vi "Getting Started - External Memory (Host).vi"() -> ()   [LabVIEW 2023]
doc: "This Host vi controls the data the flows into and out of the different external memory access methods on the FPGA."
uses:
  <vilib>/userDefined/Silver/nirio_resource_slv.ctl
  <vilib>/FPGAPlugInAG/PXIe-7966R/niLvFpga_Open_PXIe-7966R.vi
  <vilib>/rvi/interface/common/dynamic/niFpgaDynamicAddResources.vi
  <vilib>/Utility/error.llb/Error Cluster From Error Code.vi
  <vilib>/rvi/errors/niLvFpgaAdjustHostInterfaceError.vi
  <vilib>/FPGAPlugInAG/Dynamic/niLvFpga_Close_Dynamic.vi
  <vilib>/rvi/interface/nirviOpenFPGA/nirviOpenFPGA.xnode
  FPGA Bitfiles/Ext_Mem 7966R.lvbitx
  <vilib>/rvi/interface/nirviReadWriteControl/nirviReadWriteControl.xnode
  <vilib>/rvi/interface/nirviMethod/nirviMethod.xnode
  <vilib>/rvi/interface/nirviCloseFPGA/nirviCloseFPGA.xnode
  <vilib>/rvi/interface/Simulation/niFpgaSimulationCallBeginRW.vi
  <vilib>/rvi/errors/niLvFpgaMergeErrorWithErrorCode.vi
  NiFpgaLv.dll
  <vilib>/FPGAPlugInAG/Dynamic/niLvFpga_WriteFifo_Dynamic.vi
  <vilib>/FPGAPlugInAG/Dynamic/niLvFpga_ReadFifo_Dynamic.vi
panel:
  in  "Tab Control":T1(tab)
  in  "Memory Primitive - Write Address":u32
  in  "Memory Primitive - Write Data":u64
  in  "Memory Primitive - Write Valid":bool
  in  "Memory Primitive - Request Address":u32
  in  "Memory Primitive - Request Valid":bool
  out "Memory Primitive- Retrieved Data":u64
  out "Memory IDL - Retrieved Data":u64[](array[numeric])
  in  "Memory IDL - write grant time (clocks)":u16=100
  in  "Memory IDL - read grant time (clocks)":u16=100
  in  "Memory IDL - Write Data":u64[](array[numeric])
  in  "Memory IDL - Request Address":u32
  in  "Memory IDL - Request Valid":bool
  in  "Memory IDL - Write Valid":bool
  in  "Memory IDL - Write Address":u32
  in  "DRAM FIFO - Write Valid":bool
  in  "DRAM FIFO - write grant time (clocks)":u16=100
  in  "DRAM FIFO - read grant time (clocks)":u16=100
  out "DRAM FIFO Status":T2
  in  "DRAM FIFO - Write Data":u32[](array[numeric])
  out "DRAM FIFO - Retrieved Data":u32[](array[numeric])
  in  "Stop Button":bool
  in  "RIO Device":T3
  # "Overview: Demonstratethe different methods vailable for DRAM access on a FlexRIO FPGA Module.\nRequirements: LabVIEW FPGA Module, FlexRIO\nInstructions: \n 1. On the block diagram, configure the Open FPGA VI Reference function. \n 2. Return to the front panel and specify a valid RIO Device.\n 3. Run the VI \n 4. Select a tab and specify the value of Write Data  and Write address if applicable then click Write Valid.\n 5. Specify a Request Address if applicable and click Request Valid\n 6. (optional) Change the write/read grant time to zero for the read or write and observe access behavior"
  # "Note: 795x targets can read and write only the 0th element of the Write or Retrieved Data array. 796x targets the first two elements."
  # "Note: 795x targets can read and write only the first two element of the Write or Retrieved Data array.  The 796x the first four. The 797x all eight."
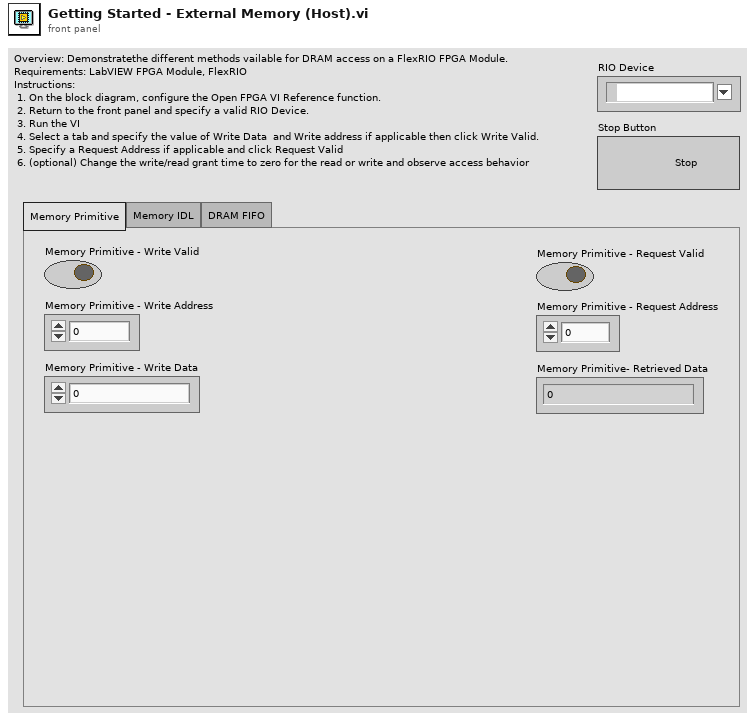
[diagram p1: front panel]
types:
  T1 = enum32{"Memory Primitive", "Memory IDL", "DRAM FIFO"}
  T2 = cluster{"Elements in To DRAM Queue":u32, "Elements in From DRAM Queue":u32, "Elements in DRAM":u32, "DRAM Full":bool, "DRAM Empty":bool}
  T3 = typedef "nirio_resource_slv.ctl" = tag
  T4 = cluster{"elements in 'to DRAM queue'":u32, "elements in 'from DRAM queue'":u32, "elements in DRAM":u32, "DRAM full":bool, "DRAM empty":bool}
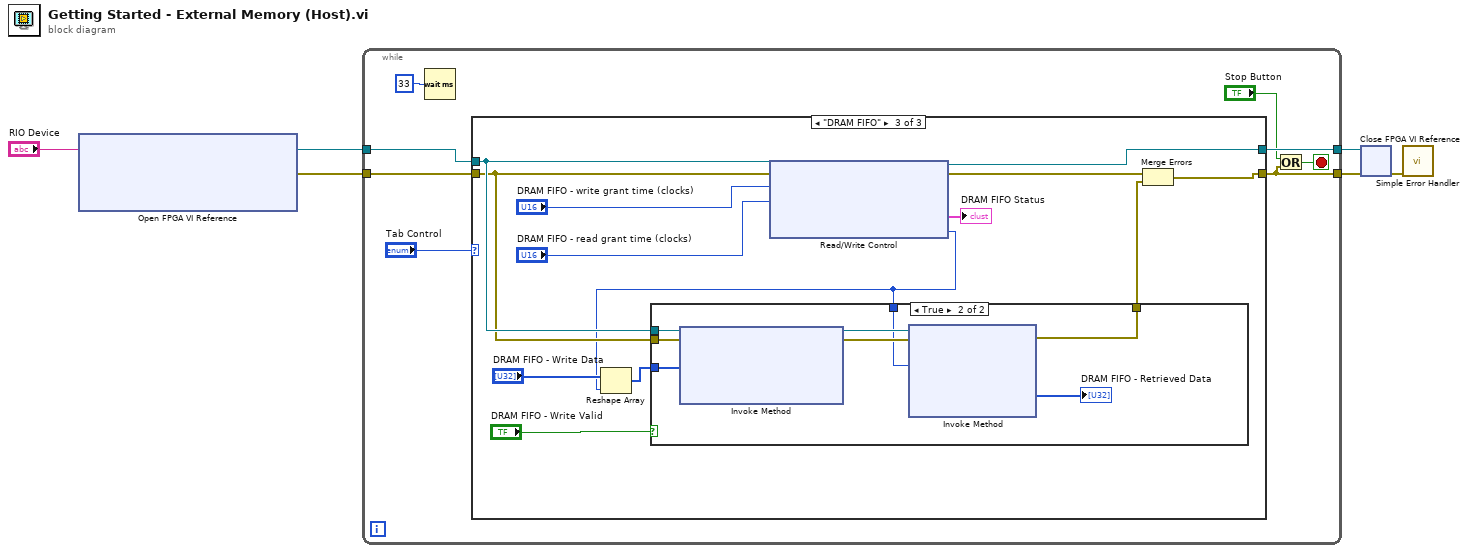
[diagram p0: block diagram]
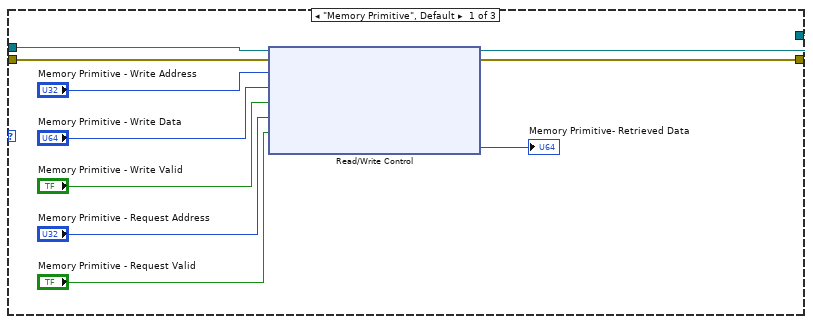
[diagram p2: hidden frame]
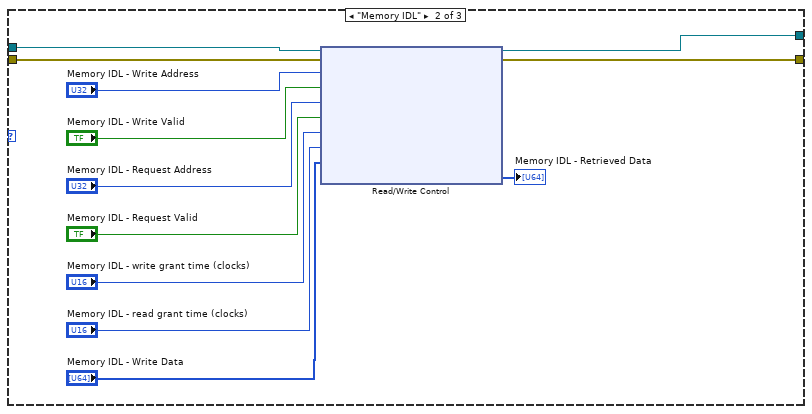
[diagram p3: hidden frame]
diagram:
  n1 = xnode "Open FPGA VI Reference"("resource name"="RIO Device") -> ("FPGA VI Reference Out"=w5:refnum<k20>, "error out"=w4:errorcluster)  [unwired: 1 in]
  n2 = while {
    tunnel: w5 -> [w14]
    tunnel: w4 -> [w12]
    tunnel: [w10] -> w2
    tunnel: [w13] -> w1
    stop <- w11 stop-if-true
    n3 = Wait (ms)(milliseconds to wait=u32 33) -> ()  [unwired: 1 out]
    n4 = case shown="\"DRAM FIFO\"" "Tab Control" {
      tunnel: w14 -> [w24 w36 w45]
      tunnel: [w23 w34 w49] -> w13
      tunnel: w12 -> [w22 w35 w44]
      tunnel: [w21 w33 w41] -> w10
      frame "Memory Primitive", Default {
        n5 = xnode "Read/Write Control"("FPGA VI Reference In"=w24, "error in"=w22, "Memory Primitive - Write Address"="Memory Primitive - Write Address", "Memory Primitive - Write Data"="Memory Primitive - Write Data", "Memory Primitive - Write Valid"="Memory Primitive - Write Valid", "Memory Primitive - Request Address"="Memory Primitive - Request Address", "Memory Primitive - Request Valid"="Memory Primitive - Request Valid") -> ("FPGA VI Reference Out"=w23:refnum<k20>, "error out"=w21:errorcluster, "Memory Primitive - Retrieved Data"=→"Memory Primitive- Retrieved Data":u64)
      }
      frame "Memory IDL" {
        n6 = xnode "Read/Write Control"("FPGA VI Reference In"=w36, "error in"=w35, "Memory IDL - Write Address"="Memory IDL - Write Address", "Memory IDL - Write Valid"="Memory IDL - Write Valid", "Memory IDL - Request Address"="Memory IDL - Request Address", "Memory IDL - Request Valid"="Memory IDL - Request Valid", "Memory IDL - write grant time"="Memory IDL - write grant time (clocks)", "Memory IDL - read grant time"="Memory IDL - read grant time (clocks)", "Memory IDL - Write Data"="Memory IDL - Write Data") -> ("FPGA VI Reference Out"=w34:refnum<k20>, "error out"=w33:errorcluster, "Memory IDL - Retrieved Data"=→"Memory IDL - Retrieved Data":u64[])
      }
      frame "DRAM FIFO" {
        n7 = xnode "Read/Write Control"("FPGA VI Reference In"=w45, "error in"=w44, "Memory IDL - write grant time"="DRAM FIFO - write grant time (clocks)", "Memory IDL - read grant time"="DRAM FIFO - read grant time (clocks)") -> ("FPGA VI Reference Out"=w49:refnum<k20>, "error out"=w42:errorcluster, "DRAM FIFO Status"=→"DRAM FIFO Status":T4, "elements per valid output"=w37:i32)
        n8 = Reshape Array("DRAM FIFO - Write Data", w37) -> (w38:u32[])
        n9 = case shown="True" "DRAM FIFO - Write Valid" {
          tunnel: w45 -> [_ w58]
          tunnel: w44 -> [w50 w57]
          tunnel: w38 -> [_ w56]
          tunnel: [w50 w52] -> w40
          tunnel: w37 -> [_ w51]
          frame False {
          }
          frame True {
            n10 = xnode "Invoke Method"("FPGA VI Reference In"=w58, "error in"=w57, "Data"=w56) -> ("FPGA VI Reference Out"=w54:refnum<k20>, "error out"=w53:errorcluster)  [unwired: 1 in, 1 out]
            n11 = xnode "Invoke Method"("FPGA VI Reference In"=w54, "error in"=w53, "Number of Elements"=w51) -> ("error out"=w52:errorcluster, "Data"=→"DRAM FIFO - Retrieved Data":u32[])  [unwired: 1 in, 2 out]
          }
        }
        n12 = Merge Errors(w42, w40) -> (w41:errorcluster)
      }
    }
    n13 = Or(x="Stop Button", y=w10) -> (x .or. y?=w11:bool)
  }
  n14 = xnode "Close FPGA VI Reference"("FPGA VI Reference In"=w1, "error in"=w2) -> ("error out"=w3:errorcluster)
  n15 = call <vilib>:"Simple Error Handler.vi"("error in (no error)"=w3) -> ()  [unwired: 4 in, 5 out]
